vi "Client TX Loop.vi"(8 "error in (no error)":errorcluster, 11 "TCPMessaging in":refnum<class "TCPMessaging.lvclass">) -> (0 "error out":errorcluster)   [LabVIEW 2020, in "Vecto.lvlib" / "TCPMessaging.lvclass"]
uses:
  TCPMessaging.lvclass
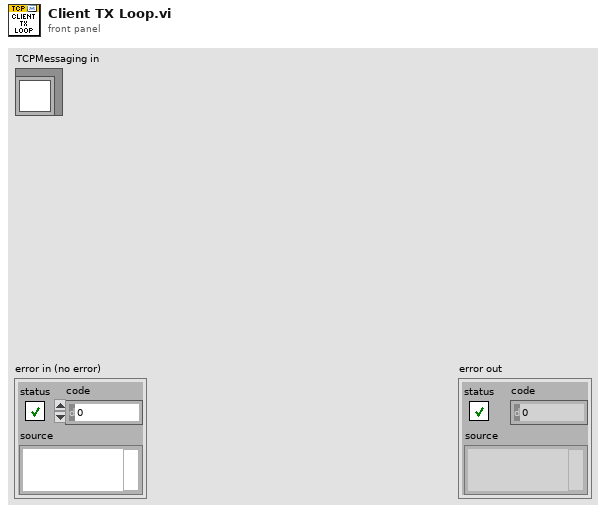
[diagram p1: front panel]
types:
  T1 = typedef "Vecto.lvlib/Send Message Data.ctl" = cluster{"TcpPayload":T2, "Register Reply":bool, "Reply Promise":refnum<class "Promise.lvclass">, "Reply Deadline":dbl}
  T2 = typedef "TcpPayload.lvlib/Data.ctl" = cluster{"target_node":u32, "target_task":u32, "source_id":u32, "sequence":u32, "timestamp":u64, "type":string, "payload":u8[]}
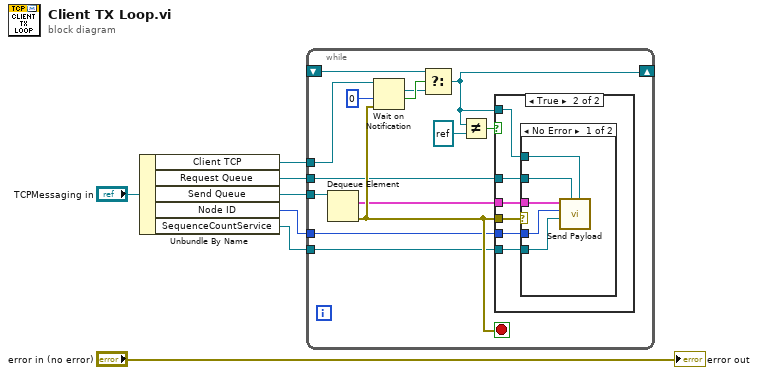
[diagram p0: block diagram]
diagram:
  n1 = Unbundle By Name("TCPMessaging in") -> ("Client TCP"=w4:refnum<notifier>, "Request Queue"=w1:refnum<queue>, "Send Queue"=w5:refnum<queue>, "Node ID"=w3:u32, "SequenceCountService"=w2:refnum<class "SequenceCountService.lvclass">)
  n2 = while {
    tunnel: w5 -> [w19]
    shift-right: [w12] -> _
    shift-left: _ -> [w16]
    tunnel: w4 -> [w15]
    tunnel: w3 -> [w10]
    tunnel: w2 -> [w9]
    tunnel: w1 -> [w8]
    stop <- w21 stop-if-true
    n3 = Dequeue Element(queue=w19) -> (element=w11:T1, error out=w21:errorcluster)  [unwired: 2 in, 2 out]
    n4 = Wait on Notification(notifier=w15, timeout in ms (-1)=0, error in (no error)=w21) -> (notification=w17:refnum<k5>, timed out?=w18:bool)  [unwired: 1 in, 2 out]
    n5 = Select(t=w16, s=w18, f=w17) -> (s? t:f=w12:refnum<k5>)
    n6 = Not Equal?(x=w12, y=refnum<k5> refnum) -> (x != y?=w13:bool)
    n7 = case shown="True" w13 {
      tunnel: w21 -> [_ w27]
      tunnel: w12 -> [_ w25]
      tunnel: w11 -> [_ w26]
      tunnel: w10 -> [_ w24]
      tunnel: w9 -> [_ w23]
      tunnel: w8 -> [_ w22]
      frame False {
        # "Not connected"
      }
      frame True {
        n8 = case shown="No Error" w27 {
          tunnel: w26 -> [w32 _]
          tunnel: w25 -> [w28 _]
          tunnel: w24 -> [w31 _]
          tunnel: w23 -> [w30 _]
          tunnel: w22 -> [w29 _]
          frame No Error {
            n9 = call "Send Payload.vi"("TCP in"=w28, "Request Queue"=w29, "SequenceCountService in"=w30, "source_id"=w31, "Send Message Data"=w32) -> ()  [unwired: 6 in, 1 out]
          }
          frame Error {
          }
        }
      }
    }
  }
  "error out" <- "error in (no error)"
